vi "ExposureDelay (SubVI).vi"(9 "Exposure Time":dbl, 10 "Exposure Start Delay in":dbl, 11 "Enum":T1(ring)) -> (3 "Exposure Start Delay out":dbl)   [LabVIEW 2023]
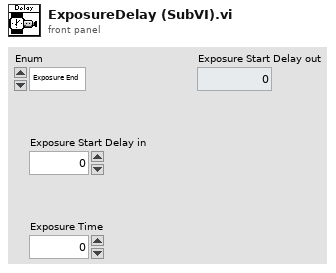
[diagram p1: front panel]
types:
  T1 = enum16{"Exposure End", "Exposure Center", "Exposure Start", "Start", "NoSync"}
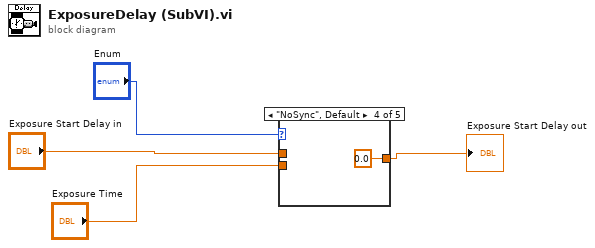
[diagram p0: block diagram]
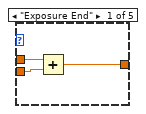
[diagram p2: hidden frame]
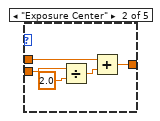
[diagram p3: hidden frame]
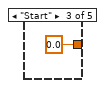
[diagram p4: hidden frame]
diagram:
  n1 = case shown="\"NoSync\", Default" "Enum" {
    tunnel: [w5 w8 0.0 0.0 w15] -> w4
    tunnel: "Exposure Start Delay in" -> [w7 w12 _ _ w15]
    tunnel: "Exposure Time" -> [w6 w11 _ _ _]
    frame "Exposure End" {
      n2 = Add(x=w7, y=w6) -> (x+y=w5:dbl)
    }
    frame "Exposure Center" {
      n3 = Divide(x=w11, y=2.0) -> (x/y=w10:dbl)
      n4 = Add(x=w12, y=w10) -> (x+y=w8:dbl)
    }
    frame "Start" {
    }
    frame "NoSync", Default {
    }
    frame "Exposure Start" {
    }
  }
  "Exposure Start Delay out" <- w4
